vi "RS_SMBV100A_Scenario_Get_Speed.vi"(6 "error in":errorcluster {"code" format="%.0x"}, 9 "Scenario info in":T2, 11 "Current Scenario Time, s":dbl) -> (0 "error out":errorcluster {"code" format="%.0x"}, 1 "scenario line out":T1, 2 "Scenario Name":string, 3 "Speed, m\\s":dbl)   [LabVIEW 2018]
uses:
  RS_SMBV100A_ScenarioInfo.ctl
  RS_SMBV100A_ScenarioLineInfo.ctl
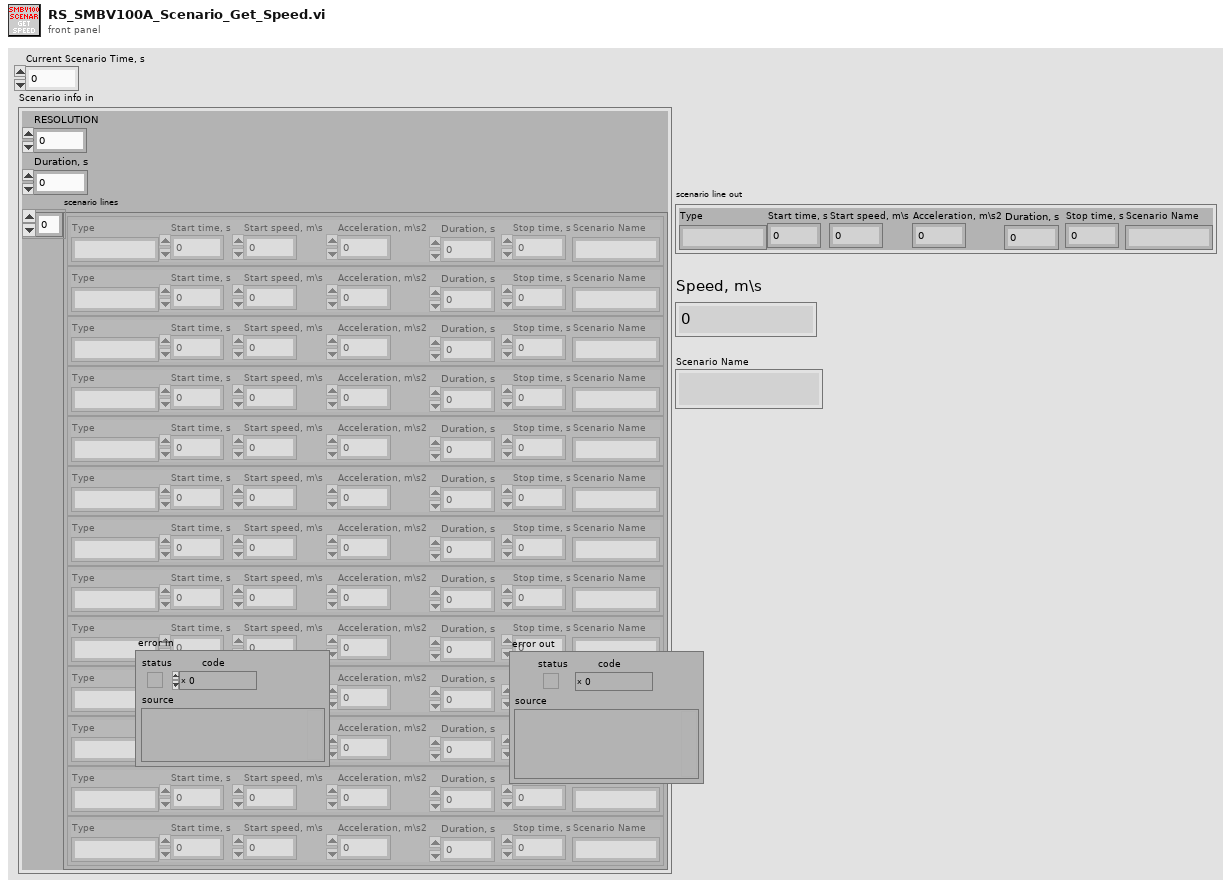
[diagram p1: front panel]
types:
  T1 = typedef "RS_SMBV100A_ScenarioLineInfo.ctl" = cluster{"Type":string, "Start time, s":dbl, "Start speed, m\\s":dbl, "Acceleration, m\\s2":dbl, "Duration, s":dbl, "Stop time, s":dbl, "Scenario Name":string}
  T2 = typedef "RS_SMBV100A_ScenarioInfo.ctl" = cluster{"RESOLUTION":dbl, "Duration, s":dbl, "scenario lines":T1[]}
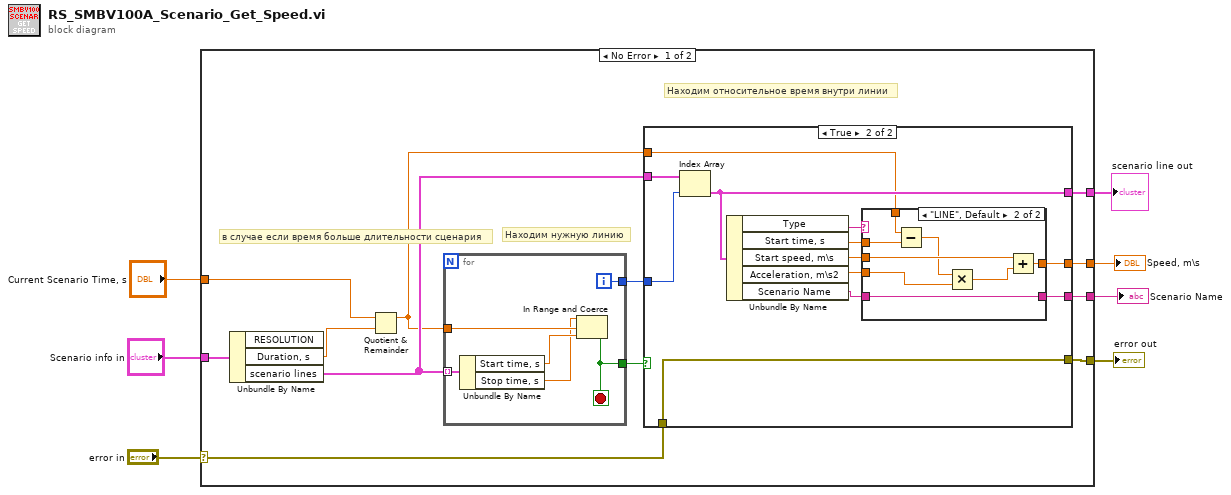
[diagram p0: block diagram]
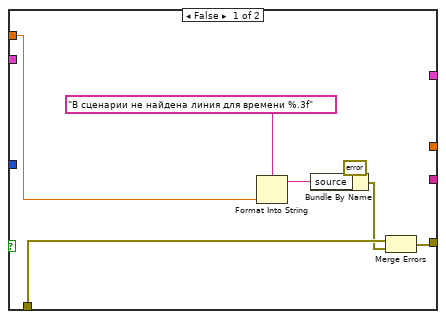
[diagram p2: hidden frame]
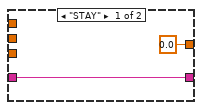
[diagram p3: hidden frame]
diagram:
  n1 = case shown="No Error" "error in" {
    selector: "error in" -> [w12 w55]
    tunnel: "Scenario info in" -> [w19 _]
    tunnel: "Current Scenario Time, s" -> [w10 _]
    tunnel: [w15 _] -> w5
    tunnel: [w14 _] -> w4
    tunnel: [w13 w55] -> w2
    tunnel: [w8 _] -> w1
    frame No Error {
      # "Находим относительное время внутри линии"
      # "Находим нужную линию"
      # "в случае если время больше длительности сценария"
      n2 = Unbundle By Name(w19) -> ("Duration, s"=w11:dbl, "scenario lines"=w16:T1[])  [unwired: 1 out]
      n3 = Quotient & Remainder(x=w10, y=w11) -> (x-y*floor(x/y)=w9:dbl)  [unwired: 1 out]
      n4 = for {
        tunnel: w16 -> [w54] mode=indexing
        tunnel: w9 -> [w53]
        tunnel: [w50] -> w17
        tunnel: [w49] -> w18
        i -> [w50]
        stop <- w49 stop-if-true
        n5 = Unbundle By Name(w54) -> ("Start time, s"=w52:dbl, "Stop time, s"=w51:dbl)
        n6 = In Range and Coerce(upper limit=w51, x=w53, lower limit=w52) -> (In Range?=w49:bool)  [unwired: 1 out]
      }
      n7 = case shown="True" w18 {
        tunnel: w17 -> [_ w37]
        tunnel: w16 -> [_ w38]
        tunnel: [_ w36] -> w15
        tunnel: w9 -> [w20 w35]
        tunnel: [_ w31] -> w14
        tunnel: [w26 w29] -> w13
        tunnel: w12 -> [w25 w29]
        tunnel: [_ w28] -> w8
        frame False {
          n8 = Format Into String(format string="В сценарии не найдена линия для времени %.3f", w20) -> (resulting string=w23:string)  [unwired: 2 in, 1 out]
          n9 = Bundle By Name(cluster=errorcluster {"status"=TRUE, "code"=5450, "source"=""} ("error in"), "source"=w23) -> (w22:errorcluster)
          n10 = Merge Errors(w25, w22) -> (w26:errorcluster)
        }
        frame True {
          n11 = Index Array(array=w38, index=w37) -> (element=w36:T1)
          n12 = Unbundle By Name(w36) -> ("Type"=w30:string, "Start time, s"=w34:dbl, "Start speed, m\\s"=w32:dbl, "Acceleration, m\\s2"=w33:dbl, "Scenario Name"=w27:string)
          n13 = case shown="\"LINE\", Default" w30 {
            tunnel: w35 -> [_ w48]
            tunnel: w34 -> [_ w47]
            tunnel: w33 -> [_ w42]
            tunnel: w32 -> [_ w46]
            tunnel: [0.0 w44] -> w31
            tunnel: [w39 w41] -> w28
            tunnel: w27 -> [w39 w41]
            frame "STAY" {
            }
            frame "LINE", Default {
              n14 = Subtract(x=w48, y=w47) -> (x-y=w43:dbl)
              n15 = Multiply(x=w43, y=w42) -> (x*y=w45:dbl)
              n16 = Add(x=w46, y=w45) -> (x+y=w44:dbl)
            }
          }
        }
      }
    }
    frame Error {
    }
  }
  "Speed, m\\s" <- w4
  "scenario line out" <- w5
  "error out" <- w2
  "Scenario Name" <- w1
